vi "Manipulator Jacobian (End Effector Frame).vi"(8 "error in (no error)":errorcluster, 10 "joint positions":dbl[](array[numeric]), 11 "serial arm in":refnum<class "NI_Robotics_Serial Robot Arm.lvclass">) -> (0 "error out":errorcluster, 1 "forward kinematics":T1, 2 "jacobian":T1, 3 "serial arm out":refnum<class "NI_Robotics_Serial Robot Arm.lvclass">)   [LabVIEW 2017, in "NI_Kinematics.lvlib"]
doc: "Generates a Jacobian matrix that transforms differential velocities in joint space to the Cartesian velocity of the end effector in the coordinate frame of the end effector.\n\n<B>.m file:</B> jacobn"
uses:
  <vilib>/robotics/Kinematics/NI_Kinematics.lvlib
  <vilib>/robotics/Kinematics/Robot/NI_Robotics_Serial Robot Arm.lvclass
  <vilib>/Analysis/Matrix/Datatypes/RealMatrix.ctl
  <vilib>/Analysis/baseanly.llb/Real A x B.vi
  <vilib>/robotics/Kinematics/Link/NI_Robotics_Link.lvclass
  <vilib>/Analysis/NI_AALBase.lvlib
  <vilib>/robotics/Utilities/NI_Robotics Utilities.lvlib
  <vilib>/Analysis/Matrix/NI_Matrix.lvlib
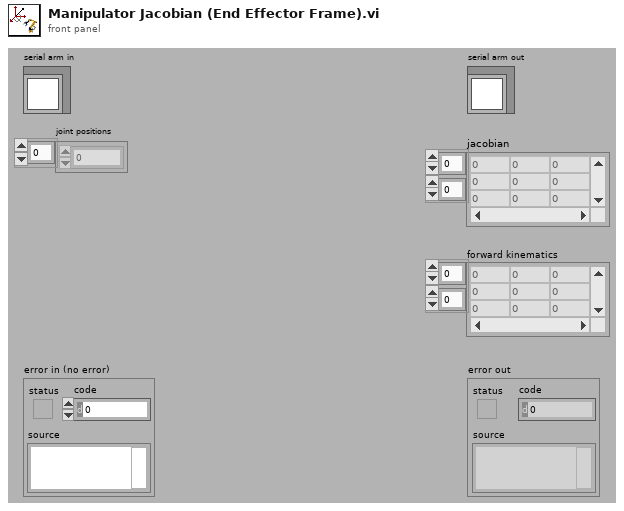
[diagram p1: front panel]
types:
  T1 = typedef "NI_Matrix.lvlib/RealMatrix.ctl" = dbl[][]
  T2 = typedef "NI_Kinematics.lvlib/DH Convention.ctl" = enum16{"Standard", "Modified"}
  T3 = typedef "NI_Robotics_Link.lvclass/Joint Type.ctl" = enum16{"Revolute", "Prismatic"}
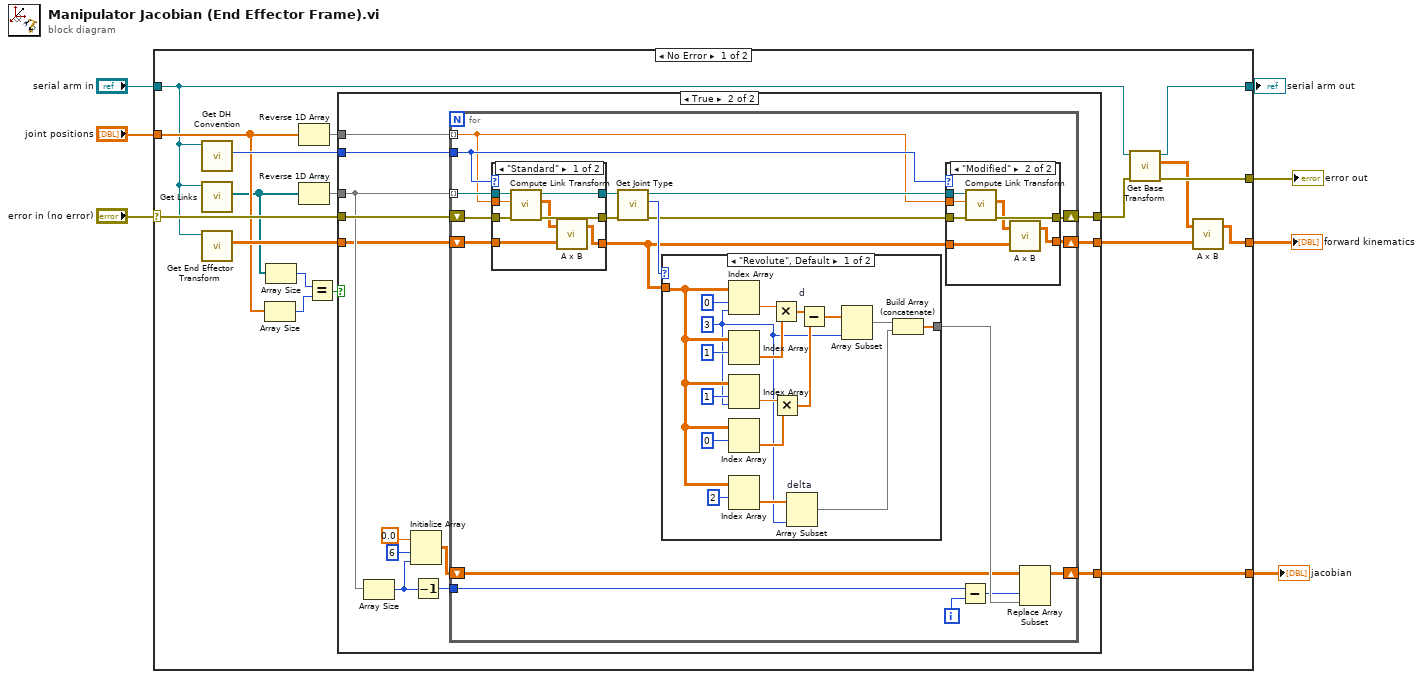
[diagram p0: block diagram]
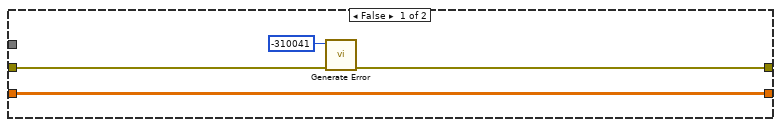
[diagram p2: hidden frame]
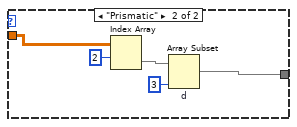
[diagram p5: hidden frame]
diagram:
  n1 = case shown="No Error" "error in (no error)" {
    selector: "error in (no error)" -> [w24 w106]
    tunnel: [w11 w106] -> w6
    tunnel: [w12 w105] -> w4
    tunnel: "serial arm in" -> [w13 w105]
    tunnel: "joint positions" -> [w19 _]
    tunnel: [w22 _] -> w2
    tunnel: [w8 _] -> w1
    frame No Error {
      n2 = call <vilib>:"Get DH Convention.vi"("serial arm in"=w13) -> ("DH Convention"=w20:T2)  [unwired: 8 in, 2 out]
      n3 = call <vilib>:"Get Links.vi"("serial arm in"=w13) -> ("links"=w18:refnum<class "NI_Robotics_Link.lvclass">[])  [unwired: 8 in, 2 out]
      n4 = call <vilib>:"Get End Effector Transform.vi"("serial arm in"=w13) -> ("end effector transform"=w21:T1)  [unwired: 8 in, 2 out]
      n5 = Array Size(array=w19) -> (size(s)=w16:i32)
      n6 = Array Size(array=w18) -> (size(s)=w17:i32)
      n7 = Reverse 1D Array(array=w19) -> (reversed array=w25:dbl[])
      n8 = Reverse 1D Array(array=w18) -> (reversed array=w23:refnum<class "NI_Robotics_Link.lvclass">[])
      n9 = Equal?(x=w17, y=w16) -> (x = y?=w15:bool)
      n10 = case shown="True" w15 {
        tunnel: w25 -> [_ w42]
        tunnel: w24 -> [w27 w41]
        tunnel: [w26 w40] -> w14
        tunnel: w23 -> [_ w37]
        tunnel: [w29 w33] -> w9
        tunnel: [_ w32] -> w22
        tunnel: w21 -> [w29 w31]
        tunnel: w20 -> [_ w30]
        frame False {
          n11 = call <vilib>:"Generate Error.vi"("error in (no error)"=w27, "code"=-310041) -> ("error out"=w26:errorcluster)  [unwired: 9 in]
        }
        frame True {
          n12 = Array Size(array=w37) -> (size(s)=w35:i32)
          n13 = Initialize Array(0.0 ("element"), 6 ("dimension size"), w35) -> (w36:dbl[][])
          n14 = Decrement(x=w35) -> (x-1=w34:i32)
          n15 = for {
            tunnel: w37 -> [w61] mode=indexing
            tunnel: w42 -> [w51] mode=indexing
            shift-right: [w49] -> w40
            shift-left: w41 -> [w60]
            shift-right: [w53] -> w33
            shift-left: w31 -> [w59]
            tunnel: w30 -> [w52]
            shift-right: [w46] -> w32
            shift-left: w36 -> [w43]
            tunnel: w34 -> [w48]
            i -> [w47]
            n16 = case shown="\"Standard\"" w52 {
              tunnel: w61 -> [w78 w81]
              tunnel: w51 -> [w77 _]
              tunnel: w60 -> [w76 w80]
              tunnel: w59 -> [w72 w79]
              tunnel: [w75 w81] -> w58
              tunnel: [w74 w80] -> w57
              tunnel: [w73 w79] -> w54
              frame "Standard" {
                n17 = call <vilib>:"Compute Link Transform.vi"("error in (no error)"=w76, "q"=w77, "Link in"=w78) -> ("error out"=w74:errorcluster, "Link Transform"=w71:T1, "Link out"=w75:refnum<class "NI_Robotics_Link.lvclass">)  [unwired: 6 out]
                n18 = call-poly <vilib>:"A x B.vi"("B"=w72, "A"=w71) -> ("A x B"=w73:T1)  [unwired: 1 out]
              }
              frame "Modified" {
              }
            }
            n19 = call <vilib>:"Get Joint Type.vi"("error in (no error)"=w57, "Link in"=w58) -> ("error out"=w50:errorcluster, "Joint Type"=w56:T3, "Link out"=w55:refnum<class "NI_Robotics_Link.lvclass">)  [unwired: 7 out]
            n20 = case shown="\"Revolute\", Default" w56 {
              tunnel: w54 -> [w89 w101]
              tunnel: [w87 w100] -> w45
              frame "Revolute", Default {
                w82 = 3 ("disabled index (col)")
                n21 = Index Array(array=w89, index (row)=0, index (col)=w82) -> (element=w95:dbl)
                n22 = Index Array(array=w89, index (row)=1) -> (element=w85:dbl[])  [unwired: 1 in]
                n23 = Index Array(array=w89, index (row)=1, index (col)=w82) -> (element=w91:dbl)
                n24 = Index Array(array=w89, index (row)=0) -> (element=w86:dbl[])  [unwired: 1 in]
                n25 = Index Array(array=w89, index (row)=2) -> (element=w99:dbl[])  [unwired: 1 in]
                n26 = Multiply ("Multiply.vi")(x=w95, y=w85) -> (x*y=w96:dbl[])
                n27 = Multiply ("Multiply.vi")(x=w91, y=w86) -> (x*y=w97:dbl[])
                n28 = Array Subset "delta"(array=w99, length=w82) -> (w88:dbl[])  [unwired: 1 in]
                n29 = Subtract "d"(x=w96, y=w97) -> (x-y=w84:dbl[])
                n30 = Array Subset(array=w84, length=w82) -> (w83:dbl[])  [unwired: 1 in]
                n31 = Build Array (concatenate)(w83, w88) -> (w87:dbl[])
              }
              frame "Prismatic" {
                n32 = Index Array(array=w101, index (row)=2) -> (element=w102:dbl[])  [unwired: 1 in]
                n33 = Array Subset "d"(array=w102, length=3) -> (w100:dbl[])  [unwired: 1 in]
              }
            }
            n34 = case shown="\"Modified\"" w52 {
              tunnel: w55 -> [_ w70]
              tunnel: w51 -> [_ w69]
              tunnel: w50 -> [w63 w68]
              tunnel: w54 -> [w62 w65]
              tunnel: [w63 w67] -> w49
              tunnel: [w62 w66] -> w53
              frame "Standard" {
              }
              frame "Modified" {
                n35 = call <vilib>:"Compute Link Transform.vi"("error in (no error)"=w68, "q"=w69, "Link in"=w70) -> ("error out"=w67:errorcluster, "Link Transform"=w64:T1)  [unwired: 7 out]
                n36 = call-poly <vilib>:"A x B.vi"("B"=w65, "A"=w64) -> ("A x B"=w66:T1)  [unwired: 1 out]
              }
            }
            n37 = Subtract(x=w48, y=w47) -> (x-y=w44:i32)
            n38 = Replace Array Subset(array=w43, new element=w45, index (col)=w44) -> (w46:dbl[][])  [unwired: 1 in]
          }
        }
      }
      n39 = call <vilib>:"Get Base Transform.vi"("error in (no error)"=w14, "serial arm in"=w13) -> ("error out"=w11:errorcluster, "base transform"=w10:T1, "serial arm out"=w12:refnum<class "NI_Robotics_Serial Robot Arm.lvclass">)  [unwired: 7 in]
      n40 = call-poly <vilib>:"A x B.vi"("B"=w9, "A"=w10) -> ("A x B"=w8:T1)  [unwired: 1 out]
    }
    frame Error {
    }
  }
  "error out" <- w6
  "serial arm out" <- w4
  "jacobian" <- w2
  "forward kinematics" <- w1
